vi "ExportConfiguration.vi"(0 "Path":path, 5 "target alias":string, 7 "Queue Name":string="Queue Name", 11 "error in (no error)":errorcluster) -> (4 "ExportedConfiguration":T1, 15 "error out":errorcluster)   [LabVIEW 2017, in "WaveformAcq runtime.lvclass"]
uses:
  WaveformAcq runtime.lvclass
  Export.ctl
  configuration/WaveformAcq configuration.lvclass
  configuration/WaveformAcq configuration.lvclass/WaveformAcq configuration.ctl
  <vilib>/NI/Configuration Framework/tree serializer/NISE_CEF_TreeSerializer.lvlib
  <vilib>/NI/DCAF/Tag Editor Core/Framework Configuration Classes/flattened data interface/PL_Serialization Interface.lvlib
  <vilib>/NI/Tag Bus Module Framework/module configuration/TBM module configuration.lvclass
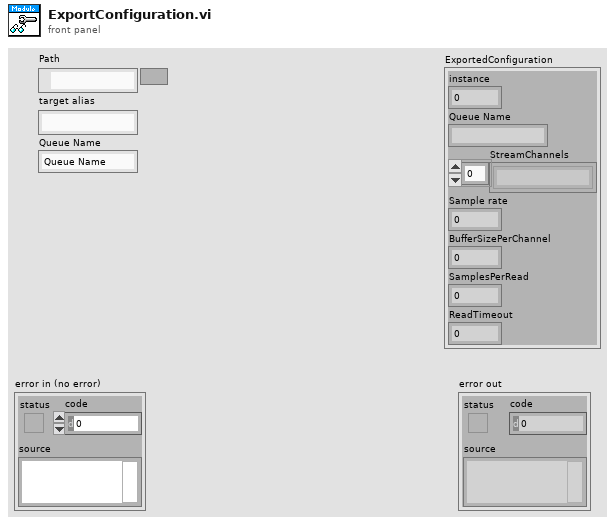
[diagram p1: front panel]
types:
  T1 = typedef "WaveformAcq runtime.lvclass/Export.ctl" = cluster{"instance":i32, "Queue Name":string, "StreamChannels":string[], "Sample rate":i32, "BufferSizePerChannel":i32, "SamplesPerRead":i32, "ReadTimeout":dbl}
  T2 = typedef "NISE_CEF_TreeSerializer.lvlib/base file format.ctl" = cluster{"version":string, "data":string}
  T3 = typedef "NISE_CEF_TreeSerializer.lvlib/flat hierarchy.ctl" = cluster{"hierarchy structure":T4, "instance data":T6[]}
  T4 = typedef "NISE_CEF_TreeSerializer.lvlib/full hierarchy.ctl" = cluster{"root":string, "hierarchy":T5[]}
  T5 = typedef "NISE_CEF_TreeSerializer.lvlib/hierarchy element.ctl" = cluster{"current node":string, "children":string[]}
  T6 = typedef "NISE_CEF_TreeSerializer.lvlib/instance data.ctl" = cluster{"ID":string, "Alias":string, "class":string, "version":string, "data":string}
  T7 = typedef "PLConfigurationSerializer.lvlib/targets cluster.ctl" = cluster{"Target Configuration":refnum<class "PL_Target Configuration.lvclass">, "engines":T8[]}
  T8 = typedef "PLConfigurationSerializer.lvlib/engines cluster.ctl" = cluster{"engine configuration":refnum<class "engine configuration.lvclass">, "modules":refnum<class "TBM module configuration.lvclass">[]}
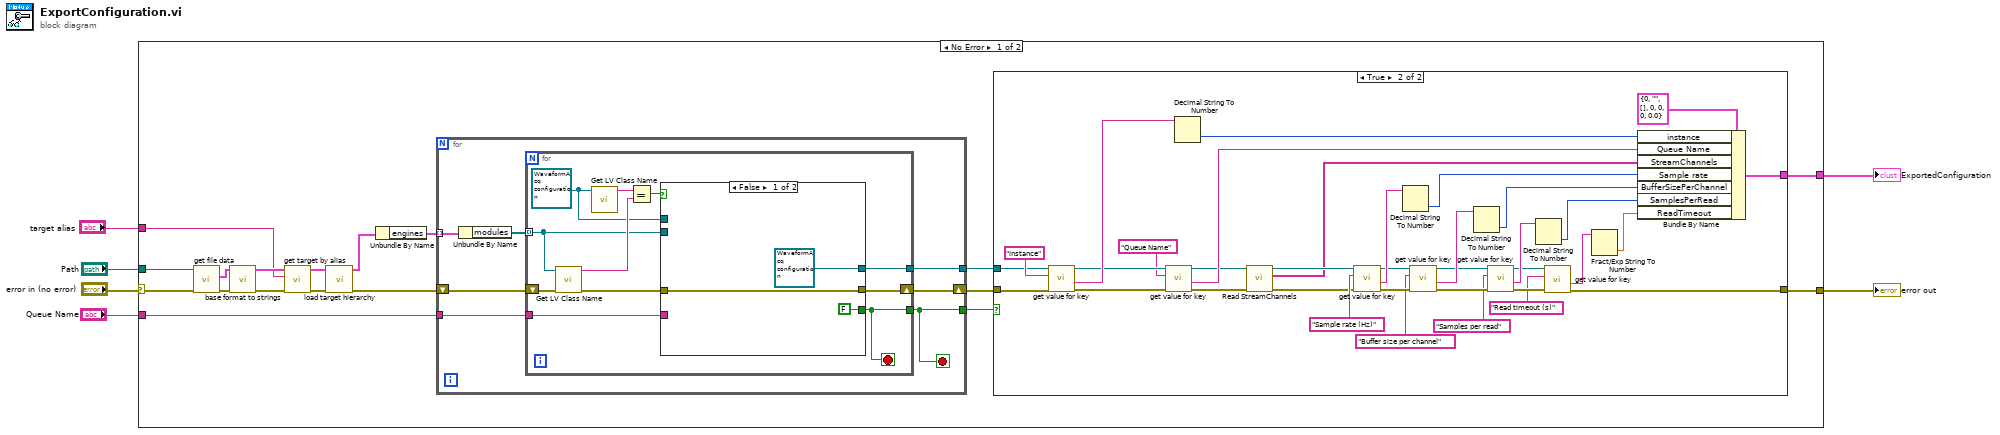
[diagram p0: block diagram]
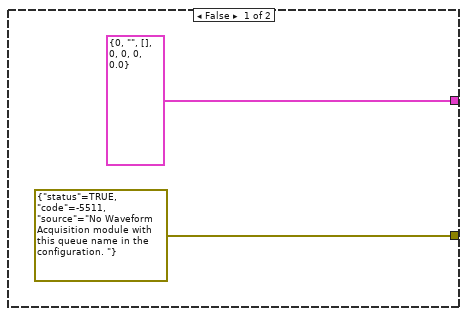
[diagram p2: hidden frame]
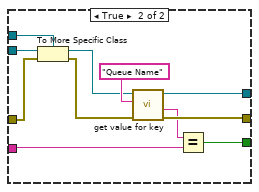
[diagram p3: hidden frame]
diagram:
  n1 = case shown="No Error" "error in (no error)" {
    selector: "error in (no error)" -> [w18 w94]
    tunnel: [w8 w94] -> w5
    tunnel: "Path" -> [w17 _]
    tunnel: "target alias" -> [w16 _]
    tunnel: "Queue Name" -> [w12 _]
    tunnel: [w7 _] -> w1
    frame No Error {
      n2 = call <vilib>:"get file data.vi"("error in"=w18, "Path"=w17) -> ("error out"=w23:errorcluster, "format"=w24:T2)  [unwired: 8 in]
      n3 = call <vilib>:"base format to strings.vi"("error in"=w23, "format"=w24) -> ("error out"=w21:errorcluster, "data"=w22:T3)  [unwired: 8 in]
      n4 = call <vilib>:"get target by alias.vi"("error in"=w21, "alias"=w16, "system hierarchy"=w22) -> ("error out"=w19:errorcluster, "target hierarchy"=w20:T3)  [unwired: 7 in]
      n5 = call <vilib>:"load target hierarchy.vi"("error in"=w19, "target hierarchy"=w20) -> ("error out"=w13:errorcluster, "targets cluster out"=w15:T7)  [unwired: 8 in]
      n6 = Unbundle By Name(w15) -> ("engines"=w14:T8[])
      n7 = for {
        tunnel: w14 -> [w68] mode=indexing
        shift-right: [w65] -> w10
        shift-left: w13 -> [w66]
        tunnel: w12 -> [w64]
        tunnel: [w63] -> w9
        tunnel: [w62] -> w11
        stop <- w62 stop-if-true
        n8 = Unbundle By Name(w68) -> ("modules"=w67:refnum<class "TBM module configuration.lvclass">[])
        n9 = for {
          tunnel: w67 -> [w75] mode=indexing
          shift-right: [w72] -> w65
          shift-left: w66 -> [w77]
          tunnel: w64 -> [w71]
          tunnel: [w70] -> w62
          tunnel: [w69] -> w63
          stop <- w70 stop-if-true
          w74 = refnum<class "WaveformAcq configuration.lvclass"> refnum ("WaveformAcq configuration")
          n10 = call <vilib>:"Get LV Class Name.vi"("error in (no error)"=w77, "object"=w75) -> ("error out"=w73:errorcluster, "class name"=w78:string)  [unwired: 8 in]
          n11 = call <vilib>:"Get LV Class Name.vi"("object"=w74) -> ("class name"=w79:string)  [unwired: 9 in, 1 out]
          n12 = Equal?(x=w79, y=w78) -> (x = y?=w76:bool)
          n13 = case shown="False" w76 {
            tunnel: w75 -> [_ w93]
            tunnel: w74 -> [_ w92]
            tunnel: w73 -> [w82 w91]
            tunnel: [w82 w87] -> w72
            tunnel: w71 -> [_ w86]
            tunnel: [FALSE w84] -> w70
            tunnel: [refnum<class "WaveformAcq configuration.lvclass"> refnum ("fixed channel configuration out") w83] -> w69
            frame False {
            }
            frame True {
              n14 = To More Specific Class(target class=w92, reference=w93, error in=w91) -> (specific class reference=w88:refnum<class "WaveformAcq configuration.lvclass">, error out=w89:errorcluster)
              n15 = call-dynamic "get value for key.vi"("error in"=w89, "key"="Queue Name" ("String"), "fixed channel configuration in"=w88) -> ("error out"=w87:errorcluster, "value"=w85:string, "fixed channel configuration out"=w83:refnum<class "WaveformAcq configuration.lvclass">)  [unwired: 6 in]
              n16 = Equal?(x=w85, y=w86) -> (x = y?=w84:bool)
            }
          }
        }
      }
      n17 = case shown="True" w11 {
        tunnel: w10 -> [_ w41]
        tunnel: w9 -> [_ w42]
        tunnel: [errorcluster {"status"=TRUE, "code"=-5511, "source"="No Waveform Acquisition module with this queue name in the configuration. "} ("error IO") w32] -> w8
        tunnel: [T1 {"instance"=0, "Queue Name"="", "StreamChannels"=[], "Sample rate"=0, "BufferSizePerChannel"=0, "SamplesPerRead"=0, "ReadTimeout"=0.0} w33] -> w7
        frame False {
        }
        frame True {
          n18 = call-dynamic "get value for key.vi"("error in"=w41, "key"="instance", "fixed channel configuration in"=w42) -> ("error out"=w50:errorcluster, "value"=w57:string, "fixed channel configuration out"=w49:refnum<class "WaveformAcq configuration.lvclass">)  [unwired: 6 in]
          n19 = call-dynamic "get value for key.vi"("error in"=w50, "key"="Queue Name" ("String"), "fixed channel configuration in"=w49) -> ("error out"=w30:errorcluster, "value"=w38:string, "fixed channel configuration out"=w31:refnum<class "WaveformAcq configuration.lvclass">)  [unwired: 6 in]
          n20 = Decimal String To Number(string=w57) -> (number=w39:i32)  [unwired: 2 in, 1 out]
          n21 = call "Read StreamChannels.vi"("error in (no error)"=w30, "WaveformAcq configuration in"=w31) -> ("error out"=w29:errorcluster, "StreamChannels"=w27:string[], "WaveformAcq configuration out"=w28:refnum<class "WaveformAcq configuration.lvclass">)  [unwired: 7 in]
          n22 = call-dynamic "get value for key.vi"("error in"=w29, "key"="Sample rate (Hz)" ("String"), "fixed channel configuration in"=w28) -> ("error out"=w53:errorcluster, "value"=w58:string, "fixed channel configuration out"=w51:refnum<class "WaveformAcq configuration.lvclass">)  [unwired: 6 in]
          n23 = Decimal String To Number(string=w58) -> (number=w37:i32)  [unwired: 2 in, 1 out]
          n24 = call-dynamic "get value for key.vi"("error in"=w53, "key"="Buffer size per channel" ("String"), "fixed channel configuration in"=w51) -> ("error out"=w54:errorcluster, "value"=w59:string, "fixed channel configuration out"=w52:refnum<class "WaveformAcq configuration.lvclass">)  [unwired: 6 in]
          n25 = Decimal String To Number(string=w59) -> (number=w36:i32)  [unwired: 2 in, 1 out]
          n26 = call-dynamic "get value for key.vi"("error in"=w54, "key"="Samples per read" ("String"), "fixed channel configuration in"=w52) -> ("error out"=w56:errorcluster, "value"=w60:string, "fixed channel configuration out"=w55:refnum<class "WaveformAcq configuration.lvclass">)  [unwired: 6 in]
          n27 = Decimal String To Number(string=w60) -> (number=w35:i32)  [unwired: 2 in, 1 out]
          n28 = call-dynamic "get value for key.vi"("error in"=w56, "key"="Read timeout (s)" ("String"), "fixed channel configuration in"=w55) -> ("error out"=w32:errorcluster, "value"=w61:string)  [unwired: 6 in, 1 out]
          n29 = Fract/Exp String To Number(string=w61) -> (number=w34:dbl)  [unwired: 3 in, 1 out]
          n30 = Bundle By Name(cluster=T1 {"instance"=0, "Queue Name"="", "StreamChannels"=[], "Sample rate"=0, "BufferSizePerChannel"=0, "SamplesPerRead"=0, "ReadTimeout"=0.0}, "instance"=w39, "Queue Name"=w38, "StreamChannels"=w27, "Sample rate"=w37, "BufferSizePerChannel"=w36, "SamplesPerRead"=w35, "ReadTimeout"=w34) -> (w33:T1)
        }
      }
    }
    frame Error {
    }
  }
  "error out" <- w5
  "ExportedConfiguration" <- w1
